vi "Init communcation.vi"(8 "error in (no error)":errorcluster, 11 "COM port":string) -> (0 "error out":errorcluster, 3 "VISA Refnum out":refnum<visa-resource-name>)   [LabVIEW 2023, in "Serial_communication.lvlib"]
uses:
  Serial_communication.lvlib
  baca436f-9238-49a7-9956-22396aaa8760.vi
  <vilib>/Instr/_visa.llb/VISA Configure Serial Port (Instr).vi
panel:
  out "Read start buffer":string
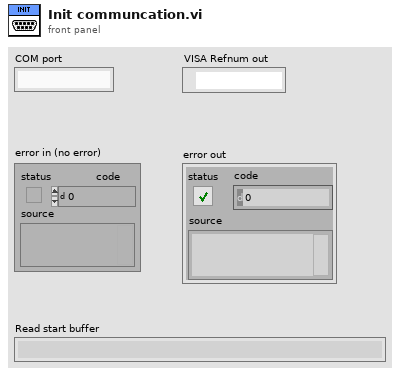
[diagram p1: front panel]
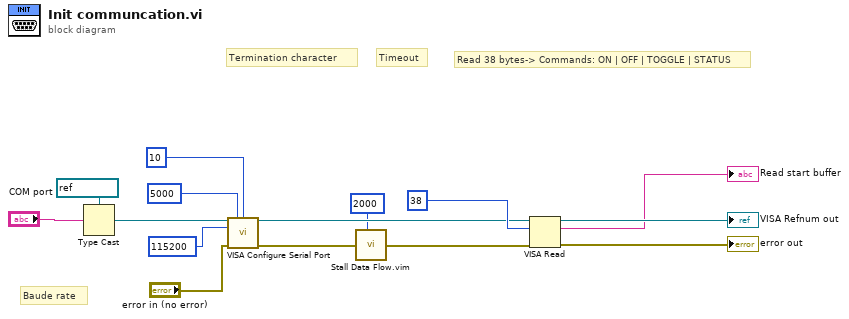
[diagram p0: block diagram]
diagram:
  # "Read 38 bytes-> Commands: ON | OFF | TOGGLE | STATUS"
  # "Baude rate"
  # "Timeout"
  # "Termination character"
  n1 = Type Cast(type=refnum<visa-resource-name> "COM5" ("VISA resource name"), x="COM port") -> (*(type *) &x=w2:refnum<visa-resource-name>)
  n2 = call-poly "VISA Configure Serial Port"("VISA resource name"=w2, "timeout (10sec)"=u32 5000, "termination char\n(0xA = '\\n' = LF)"=u8 10 ("termination char\n(0xA = '\\n' = LF)"), "baud rate (9600)"=u32 115200, "error in (no error)"="error in (no error)") -> ("VISA resource name out"=w8:refnum<visa-resource-name>, "error out"=w7:errorcluster)  [unwired: 9 in]
  n3 = call "Stall Data Flow.vim"("value in"=w7, "milliseconds to wait"=u32 2000) -> ("value out"=w5:errorcluster)  [unwired: 1 out]
  n4 = VISA Read(VISA resource name=w8, byte count=u32 38, error in (no error)=w5) -> (VISA resource name out=→"VISA Refnum out":refnum<visa-resource-name>, read buffer=→"Read start buffer":string, error out=→"error out":errorcluster)  [unwired: 1 out]
